vi "Surrounding Positions.vi"() -> ()   [LabVIEW 2018]
panel:
  out "array w/ subset deleted":cluster{"W":i32, "Z":i32, "Y":i32, "X":i32}[](array[cluster])
  in  "W":i32
  in  "X":i32
  in  "Y":i32
  in  "Z":i32
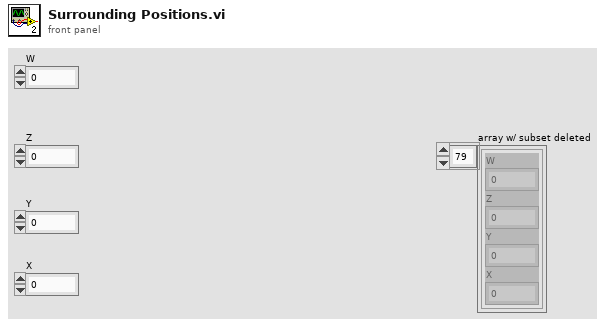
[diagram p1: front panel]
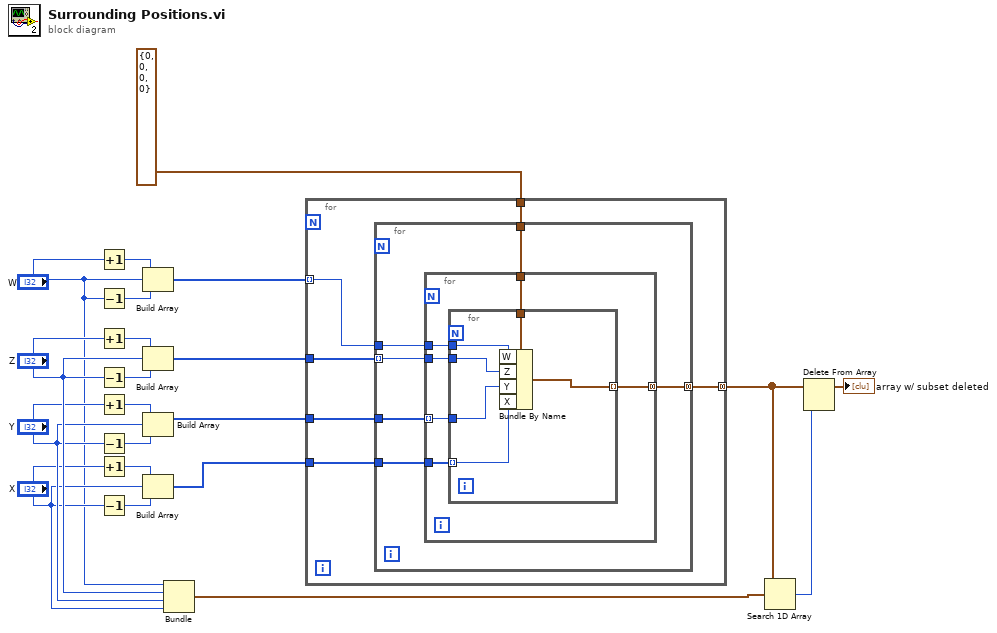
[diagram p0: block diagram]
diagram:
  n1 = Increment(x="W") -> (x+1=w7:i32)
  n2 = Decrement(x="W") -> (x-1=w8:i32)
  n3 = Increment(x="Z") -> (x+1=w21:i32)
  n4 = Decrement(x="Z") -> (x-1=w20:i32)
  n5 = Increment(x="Y") -> (x+1=w17:i32)
  n6 = Decrement(x="Y") -> (x-1=w18:i32)
  n7 = Increment(x="X") -> (x+1=w16:i32)
  n8 = Decrement(x="X") -> (x-1=w15:i32)
  n9 = Build Array(w7, "W", w8) -> (w2:i32[])
  n10 = Build Array(w21, "Z", w20) -> (w19:i32[])
  n11 = Build Array(w17, "Y", w18) -> (w6:i32[])
  n12 = Build Array(w16, "X", w15) -> (w5:i32[])
  n13 = Bundle("W"="W", "Z"="Z", "Y"="Y", "X"="X") -> (w4:cluster{"W":i32, "Z":i32, "Y":i32, "X":i32})  [unwired: 1 in]
  n14 = for {
    tunnel: w19 -> [w27]
    tunnel: [w26] -> w11 mode=concatenating
    tunnel: cluster{"W":i32, "Z":i32, "Y":i32, "X":i32} {"W"=0, "Z"=0, "Y"=0, "X"=0} -> [w25]
    tunnel: w6 -> [w24]
    tunnel: w5 -> [w23]
    tunnel: w2 -> [w22] mode=indexing
    n15 = for {
      tunnel: w27 -> [w31] mode=indexing
      tunnel: w24 -> [w33]
      tunnel: w23 -> [w32]
      tunnel: [w30] -> w26 mode=concatenating
      tunnel: w25 -> [w29]
      tunnel: w22 -> [w28]
      n16 = for {
        tunnel: w33 -> [w37] mode=indexing
        tunnel: w32 -> [w39]
        tunnel: w31 -> [w38]
        tunnel: [w36] -> w30 mode=concatenating
        tunnel: w29 -> [w35]
        tunnel: w28 -> [w34]
        n17 = for {
          tunnel: w39 -> [w44] mode=indexing
          tunnel: w38 -> [w41]
          tunnel: w37 -> [w45]
          tunnel: [w43] -> w36 mode=indexing
          tunnel: w35 -> [w42]
          tunnel: w34 -> [w40]
          n18 = Bundle By Name(cluster=w42, "W"=w40, "Z"=w41, "Y"=w45, "X"=w44) -> (w43:cluster{"W":i32, "Z":i32, "Y":i32, "X":i32})
        }
      }
    }
  }
  n19 = Search 1D Array(1D array=w11, element=w4) -> (index of element=w10:i32)  [unwired: 1 in]
  n20 = Delete From Array(array=w11, index=w10) -> (array with subset deleted=→"array w/ subset deleted":cluster{"W":i32, "Z":i32, "Y":i32, "X":i32}[])  [unwired: 1 in, 1 out]
